vi "DSF.Transceiver.UDP.Errors.vi"   [LabVIEW 2017, in "DSF.Transceiver.UDP.lvlib" / "DSF.Transceiver.UDP.lvclass"]
uses:
  DSF.Transceiver.UDP.lvclass
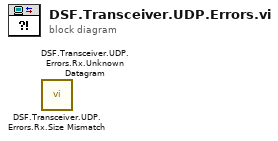
[diagram p0: block diagram]
diagram:
  n1 = call "DSF.Transceiver.UDP.Errors.Rx.Size Mismatch.vi"() -> ()  [unwired: 10 in, 2 out]
  n2 = call "DSF.Transceiver.UDP.Errors.Rx.Unknown Datagram.vi"() -> ()  [unwired: 10 in, 2 out]
